vi "Load EEPROM Data.vi"(8 "error in (no error)":errorcluster, 11 "State-machine Local Variables":T1={"Message"="", "Homed?"=FALSE, "NextState"=enum."Timeout", "G.Load"=0.0, "G.Position"=0.0, "Load#"=0, "[G.Loads]"=[], "[TotalLoads]"=[], "[Errors]"=[], "ZeroWait"=0, "Results"=[], "DwellWait"=FALSE, "Test Result"=FALSE, "[CondyleLoads]"=[], "[Max]"=[], "[Min]"=[], "Valid String?"=FALSE, "ScanTime"=timestamp(0 s since 1904-01-01), "ScannedString"="", "LabelDevID"=0, "MfgDate"=timestamp(0 s since 1904-01-01), "[EEPROM Cmds]"=[], "[CalData]"=[], "[A/Ds]"=[], "[A/Dmax]"=[], "[A/Dmin]"=[], "BattMax"=0.0, "BattMin"=0.0, "DwellTime"=2000, "PendingDeviceType"="", "Zero G.load"=0.0, "GAINC Value"="", "Programming Step"=enum."Load EEPROM", "Front Panel Program?"=FALSE, "Final Program?"=FALSE, "PCB Score"=100, "AssyScore"=100, "Pass/Fail #"="", "Result String"="", "Programming Mode"=enum."Initial Program", "Angle Test Step"=enum."Initialize", "Accel Values"=[], "Shutdown Counter"=0, "V1"=0, "V2"=0, "V3"=0, "V4"=0, "EEPROM Data"=[], "Counter"=0, "Page#"=0, "Timer"=timestamp(0 s since 1904-01-01), "Use Mark10?"=FALSE, "Eng-Result#"=0, "DUT Serial #"=0, "Scroll Message?"=FALSE, "Clear Message"=FALSE, "Batt Test Step "=enum."Initialize", "RXTX Window Found?"=FALSE, "Shutdown First Call?"=FALSE, "A2 Delay (msec)"=500, "Support Script"={"Script #"="", "Script Revision"="", "[OEMs]"=[], "[[DeviceTypes]]"=[], "[[DeviceTypesVals]]"=[], "[[List of Errors]]"=[], "Default GAINC"="", "[[ASICtrims]]"=[], "ID For Echo"="", "Condyle A CalFactor"=100, "Condyle B CalFactor"=100, "[OEMs Prefix]"=[], "Packet ID 18"="", "[[Force Table Load Test]]"=[], "[[Force Table AccurTest]]"=[]}, "Serial Table"={"Serial File Path"=path "", "[[Serial Lookup Table]]"=[], "Serial Device Info"=[], "Valid Serial?"=FALSE}, "Target Information"={"Target Brand"="", "Target DeviceType"="", "Target Serial#"=100, "Target Lot#"=0, "Target DevID"=0, "Target Channel"=5}, "Operator"="", "COM Port"="", "Config Path"=path "", "Tx Array"=[], "DUT Parameters"={"Channel"=0, "DeviceID"=0, "Script Rev"=0, "Month"=0, "Day"=0, "Year"=0, "Lot#"=0, "V1"=0, "V2"=0, "V3"=0, "V4"=0, "MFG"=0, "Cal FactorA 10"=0, "Cal FactorB 10  "=0, "Cal FactorA 16"=0, "Cal FactorB 16"=0, "ASICtrim"=[], "TmpChan"=0, "GAINC"="", "Brand"="", "Device"="", "Serial #"=0, "Batt310"=0, "Batt 280"=0}, "FTS Main?"=FALSE, "Loading"={"[Forces]"=[], "[Dwell]"=[], "Loading Step"=enum."Initialize Test"}, "Software Version"="", "Correction Factor"="", "Second Load Test"=FALSE, "Acc Loads"=[], "Mark10 Config"={"H2S%"=[80.0, 85.0, 90.0, 95.0, 100.0], "H2S Speed"=[12.0, 8.0, 6.0, 4.0, 2.0], "H to S"=2.0, "Home Speed"=1.0, "LoadWin"=0.0, "Load Speed"=0.0, "PID"={"Kp"=0.04, "Kd"=0.005001, "Ki"=2.9999999999999923e-05}}, "Channels"={"Transceiver Ch"=5, "Operating Ch"=5, "Start Ch"=0}, "Channel EEPROM"=[], "Load Notes"=[], "Engr Log?"=FALSE, "Time"=[], "Program Retry"=FALSE, "Operator Channel"="", "Target Channel "="", "New Data Program"=FALSE, "NFHU Pass?"=FALSE, "Cycle Number"=0, "Cal Cycle#"=0, "[Avg G.Loads] "=[], "[Avg A/Ds] "=[], "Cal Retry?"=FALSE, "[Total A/Ds]  "=[], "Cycle Num LA"=0, "LA Cycle# "=0, "Shim Num"=0, "Shim#  "=0, "Angle Test?"=FALSE} {"Mark10 Config"."PID"."Ki" min=0.0 max=200.0 format="%.6f"; "Mark10 Config"."PID"."Kd" min=0.0 max=200.0 format="%.6f"; "Mark10 Config"."PID"."Kp" min=0.0 max=200.0 format="%.6f"; "DUT Parameters"."ASICtrim" format="%02x"}) -> (0 "error out":errorcluster, 3 "EEPROM data":u8[][](array[numeric]) format="%02x")   [LabVIEW 2015]
uses:
  Controls/LocalVars.ctl
  Controls/Gen2 FT states.ctl
  Controls/Iniial Device Programming.ctl
  SubVI/ProgramStageControl.ctl
  Controls/Batt Cap Steps.ctl
  Controls/Support Script.ctl
  Controls/Serial Table.ctl
  Controls/Device Information.ctl
  Controls/InfoPacket.ctl
  Controls/Loading.ctl
  Controls/Load Step.ctl
  Controls/Mark10 Config.ctl
  Controls/PID parameters.ctl
  Controls/Channels.ctl
  Controls/DevEEPROMstates.ctl
  <vilib>/Utility/NIReport.llb/NI_report.lvclass
  <vilib>/addons/_office/excel.llb/Excel Get Data ([str]).vi
  <vilib>/addons/_office/NI_ReportGenerationToolkit.lvlib
  <vilib>/Utility/NIReport.llb/Excel/NI_Excel.lvclass
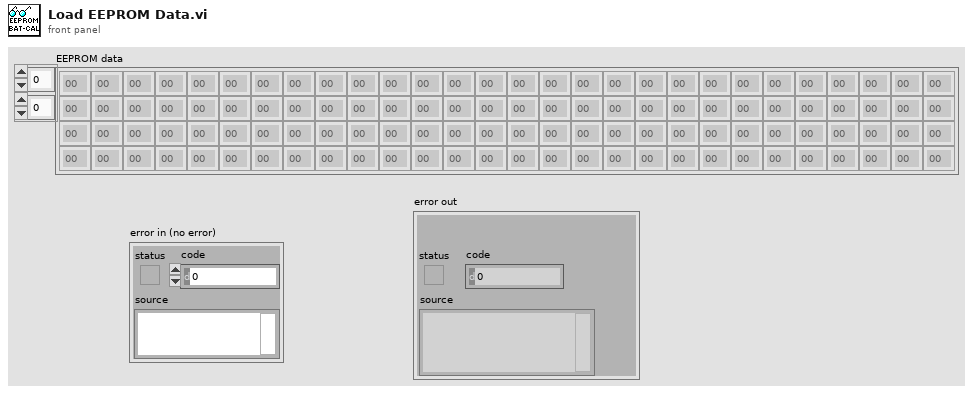
[diagram p1: front panel]
types:
  T1 = typedef "LocalVars.ctl" = cluster{"Message":string, "Homed?":bool, "NextState":T2, "G.Load":dbl, "G.Position":dbl, "Load#":i32, "[G.Loads]":dbl[], "[TotalLoads]":dbl[], "[Errors]":dbl[][], "ZeroWait":u32, "Results":dbl[], "DwellWait":bool, "Test Result":bool, "[CondyleLoads]":dbl[][], "[Max]":dbl[], "[Min]":dbl[], "Valid String?":bool, "ScanTime":timestamp, "ScannedString":string, "LabelDevID":u32, "MfgDate":timestamp, "[EEPROM Cmds]":u8[][], "[CalData]":u8[][], "[A/Ds]":dbl[][], "[A/Dmax]":dbl[], "[A/Dmin]":dbl[], "BattMax":dbl, "BattMin":dbl, "DwellTime":i32, "PendingDeviceType":string, "Zero G.load":dbl, "GAINC Value":string, "Programming Step":T3, "Front Panel Program?":bool, "Final Program?":bool, "PCB Score":i32, "AssyScore":i32, "Pass/Fail #":string, "Result String":string, "Programming Mode":T4, "Angle Test Step":enum16{"Initialize", "Get X", "Get Y", "Get Z", "Next Test"}, "Accel Values":dbl[][], "Shutdown Counter":u32, "V1":i32, "V2":i32, "V3":i32, "V4":i32, "EEPROM Data":i32[][], "Counter":i32, "Page#":i32, "Timer":timestamp, "Use Mark10?":bool, "Eng-Result#":u32, "DUT Serial #":i32, "Scroll Message?":bool, "Clear Message":bool, "Batt Test Step ":T5, "RXTX Window Found?":bool, "Shutdown First Call?":bool, "A2 Delay (msec)":i16, "Support Script":T6, "Serial Table":T7, "Target Information":T8, "Operator":string, "COM Port":string, "Config Path":path, "Tx Array":u8[], "DUT Parameters":T9, "FTS Main?":bool, "Loading":T10, "Software Version":string, "Correction Factor":string, "Second Load Test":bool, "Acc Loads":dbl[][], "Mark10 Config":T12, "Channels":T14, "Channel EEPROM":i32[][], "Load Notes":string[], "Engr Log?":bool, "Time":timestamp[], "Program Retry":bool, "Operator Channel":string, "Target Channel ":string, "New Data Program":bool, "NFHU Pass?":bool, "Cycle Number":i32, "Cal Cycle#":i32, "[Avg G.Loads] ":dbl[], "[Avg A/Ds] ":dbl[][], "Cal Retry?":bool, "[Total A/Ds]  ":dbl[][], "Cycle Num LA":i32, "LA Cycle# ":i32, "Shim Num":i32, "Shim#  ":i32, "Angle Test?":bool}
  T2 = typedef "Gen2 FT states.ctl" = enum16{"---------SETUP-------", "Initialization", "Read Support Data", "Initialize Mark-10", "Initialize Transceiver", "------UTILITIES------", "Change DUT Channel", "Find RxTx Window", "Reset Device", "Scan Channels", "Read Serial Lookup", "Shutdown Device", "ESTOP", "--------USER---------", "Timeout", "-----PROGRAM-----", "Program Device", "------MARK10--------", "Go Home", "MoveUp", "MoveDown", "Goto Load", "Goto Position", "Stop Motor", "---------TESTS--------", "Start Test", "Angle Test", "Load Test", "Load Accuracy Test", "Battery Test", "------RESULTS-------", "End Test", "Display Result", "--------EXIT--------", "Exit"}
  T3 = typedef "Iniial Device Programming.ctl" = enum16{"Load EEPROM", "Send First A1", "Send EEPROM", "Send A1", "Check EEPROM Echo", "Verify transmission", "Programming Successful", "Programming Failed"}
  T4 = typedef "ProgramStageControl.ctl" = enum16{"Initial Program", "GainC", "Scales"}
  T5 = typedef "Batt Cap Steps.ctl" = enum16{"Initialize", "Collect 2.8 Volts", "Collect 3.1 Volts", "Check Results"}
  T6 = typedef "Support Script.ctl" = cluster{"Script #":string, "Script Revision":string, "[OEMs]":string[], "[[DeviceTypes]]":string[][], "[[DeviceTypesVals]]":u16[][], "[[List of Errors]]":string[][], "Default GAINC":string, "[[ASICtrims]]":u8[][], "ID For Echo":string, "Condyle A CalFactor":i32, "Condyle B CalFactor":i32, "[OEMs Prefix]":string[], "Packet ID 18":string, "[[Force Table Load Test]]":dbl[][], "[[Force Table AccurTest]]":dbl[][]}
  T7 = typedef "Serial Table.ctl" = cluster{"Serial File Path":path, "[[Serial Lookup Table]]":string[][], "Serial Device Info":string[], "Valid Serial?":bool}
  T8 = typedef "Device Information.ctl" = cluster{"Target Brand":string, "Target DeviceType":string, "Target Serial#":i32, "Target Lot#":u32, "Target DevID":u32, "Target Channel":u8}
  T9 = typedef "InfoPacket.ctl" = cluster{"Channel":u8, "DeviceID":u32, "Script Rev":u8, "Month":u8, "Day":u8, "Year":u8, "Lot#":u32, "V1":u16, "V2":u16, "V3":u16, "V4":u16, "MFG":u8, "Cal FactorA 10":u8, "Cal FactorB 10  ":u8, "Cal FactorA 16":u8, "Cal FactorB 16":u8, "ASICtrim":u8[], "TmpChan":u8, "GAINC":string, "Brand":string, "Device":string, "Serial #":u64, "Batt310":u16, "Batt 280":u16}
  T10 = typedef "Loading.ctl" = cluster{"[Forces]":dbl[], "[Dwell]":dbl[], "Loading Step":T11}
  T11 = typedef "Load Step.ctl" = enum16{"Initialize Test", "Go Home", "Detect Dev Surface", "Wait to zero Device", "Zero Device", "Do Test", "Test Result"}
  T12 = typedef "Mark10 Config.ctl" = cluster{"H2S%":dbl[], "H2S Speed":dbl[], "H to S":dbl, "Home Speed":dbl, "LoadWin":dbl, "Load Speed":dbl, "PID":T13}
  T13 = typedef "PID parameters.ctl" = cluster{"Kp":dbl, "Kd":dbl, "Ki":dbl}
  T14 = typedef "Channels.ctl" = cluster{"Transceiver Ch":u8, "Operating Ch":u8, "Start Ch":u8}
  T15 = typedef "DevEEPROMstates.ctl" = enum16{"Open Template", "Setup parameters", "Inject parameters", "Read EEPROM data", "Close Template"}
  T16 = enum16{"maximized", "minimized", "normal", "no change"}
  T17 = enum16{"Standard Report", "HTML", "Word", "Excel"}
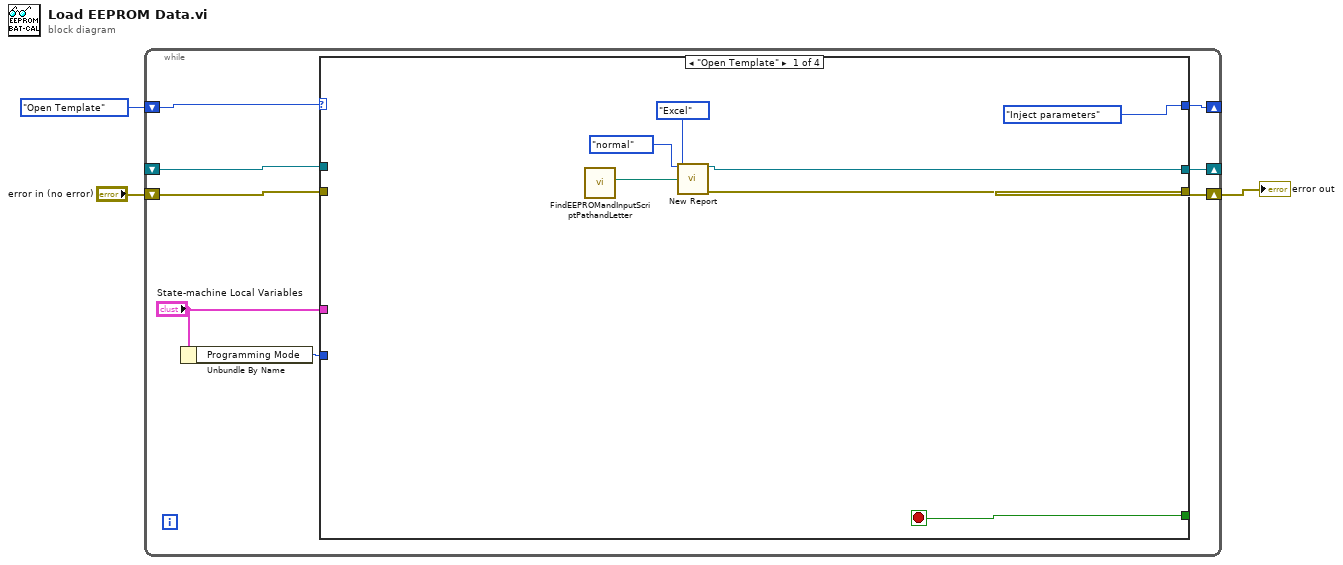
[diagram p0: block diagram]
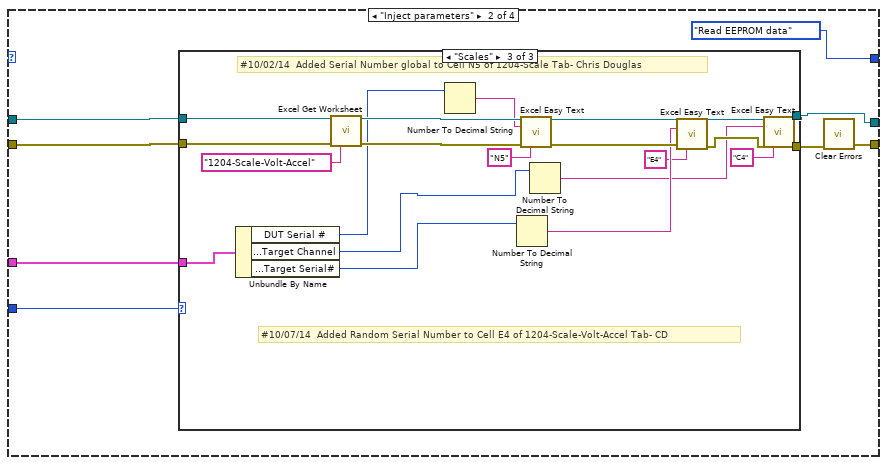
[diagram p2: hidden frame]
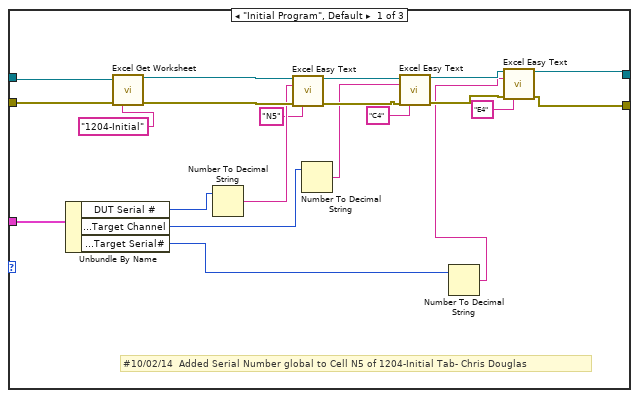
[diagram p3: hidden frame]
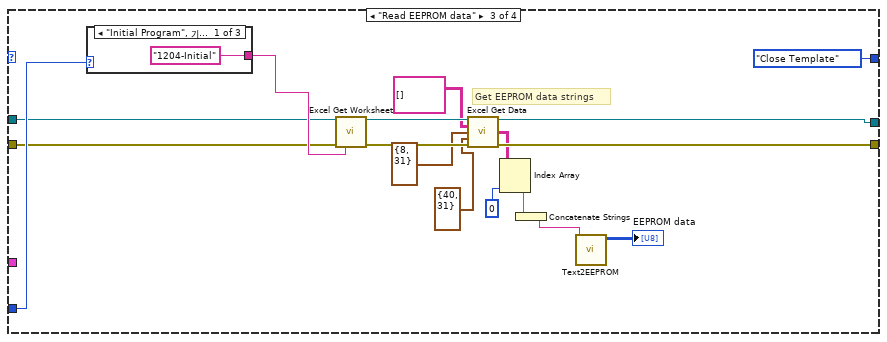
[diagram p5: hidden frame]
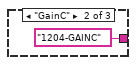
[diagram p6: hidden frame]
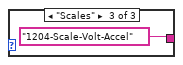
[diagram p7: hidden frame]
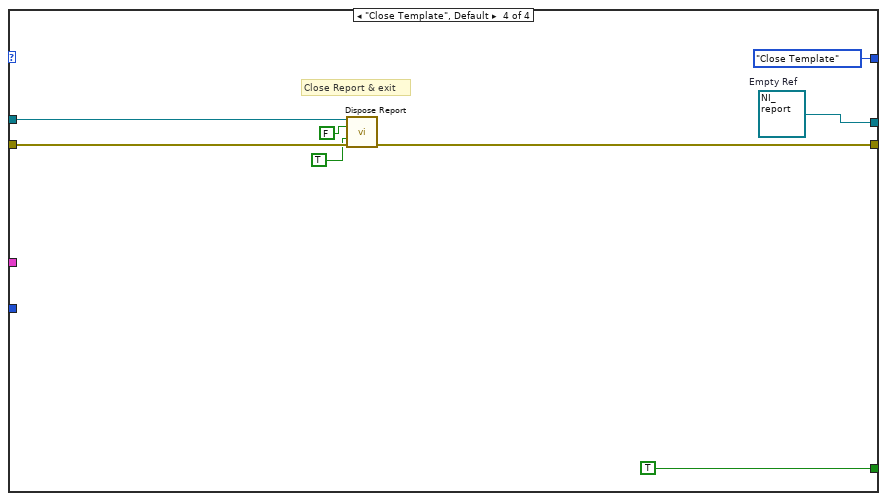
[diagram p8: hidden frame]
diagram:
  n1 = while {
    shift-right: [w4] -> _
    shift-left: _ -> [w11]
    shift-right: [w10] -> w2
    shift-left: "error in (no error)" -> [w9]
    shift-right: [w5] -> _
    shift-left: DevEEPROMstates."Open Template" -> [w8]
    stop <- w12 stop-if-true
    n2 = Unbundle By Name("State-machine Local Variables") -> ("Programming Mode"=w7:T4)
    n3 = case shown="\"Open Template\"" w8 {
      tunnel: [_ _ _ TRUE] -> w12
      tunnel: w11 -> [_ w26 w74 w97]
      tunnel: [w17 w24 w84 w95] -> w10
      tunnel: w9 -> [_ w25 w73 w96]
      tunnel: w7 -> [_ w22 w78 _]
      tunnel: "State-machine Local Variables" -> [_ w21 _ _]
      tunnel: [DevEEPROMstates."Inject parameters" DevEEPROMstates."Read EEPROM data" DevEEPROMstates."Close Template" DevEEPROMstates."Close Template"] -> w5
      tunnel: [w13 w19 w71 w91] -> w4
      frame "Open Template" {
        n4 = call "FindEEPROMandInputScriptPathandLetter.vi"() -> ("Engr Result Path"=w15:path)  [unwired: 7 in, 2 out]
        n5 = call <vilib>:"New Report.vi"("window state (normal)"=T16."normal", "report type"=T17."Excel", "template (empty)"=w15) -> ("report out"=w13:refnum<class "NI_report.lvclass">, "error out"=w17:errorcluster)  [unwired: 11 in]
      }
      frame "Inject parameters" {
        n6 = case shown="\"Scales\"" w22 {
          tunnel: w26 -> [w45 w49 w65]
          tunnel: w25 -> [w44 w48 w64]
          tunnel: [w29 w49 w55] -> w19
          tunnel: [w28 w48 w56] -> w23
          tunnel: w21 -> [w36 _ w53]
          frame "Initial Program", Default {
            # "#10/02/14  Added Serial Number global to Cell N5 of 1204-Initial Tab- Chris Douglas"
            n7 = Unbundle By Name(w36) -> ("DUT Serial #"=w34:i32, "Target Information.Target Channel"=w35:u8, "Target Information.Target Serial#"=w27:i32)
            n8 = call <vilib>:"Excel Get Worksheet.vi"("report in"=w45, "error in (no error)"=w44, "name (\"\")"="1204-Initial" ("name (\"\")")) -> ("report out"=w47:refnum<class "NI_report.lvclass">, "error out"=w46:errorcluster)  [unwired: 11 in]
            n9 = Number To Decimal String(number=w34) -> (decimal integer string=w42:string)  [unwired: 1 in]
            n10 = call <vilib>:"Excel Easy Text.vi"("report in"=w47, "text"=w42, "error in (no error)"=w46, "name (\"\")"="N5" ("name (\"\")")) -> ("report out"=w38:refnum<class "NI_report.lvclass">, "error out"=w39:errorcluster)  [unwired: 7 in, 3 out]
            n11 = Number To Decimal String(number=w35) -> (decimal integer string=w37:string)  [unwired: 1 in]
            n12 = call <vilib>:"Excel Easy Text.vi"("report in"=w38, "text"=w37, "error in (no error)"=w39, "name (\"\")"="C4" ("name (\"\")")) -> ("report out"=w32:refnum<class "NI_report.lvclass">, "error out"=w31:errorcluster)  [unwired: 7 in, 3 out]
            n13 = Number To Decimal String(number=w27) -> (decimal integer string=w30:string)  [unwired: 1 in]
            n14 = call <vilib>:"Excel Easy Text.vi"("report in"=w32, "text"=w30, "error in (no error)"=w31, "name (\"\")"="E4" ("name (\"\")")) -> ("report out"=w29:refnum<class "NI_report.lvclass">, "error out"=w28:errorcluster)  [unwired: 7 in, 3 out]
          }
          frame "GainC" {
          }
          frame "Scales" {
            # "#10/07/14  Added Random Serial Number to Cell E4 of 1204-Scale-Volt-Accel Tab- CD"
            # "#10/02/14  Added Serial Number global to Cell N5 of 1204-Scale Tab- Chris Douglas"
            n15 = Unbundle By Name(w53) -> ("DUT Serial #"=w51:i32, "Target Information.Target Channel"=w52:u8, "Target Information.Target Serial#"=w50:i32)
            n16 = call <vilib>:"Excel Get Worksheet.vi"("report in"=w65, "error in (no error)"=w64, "name (\"\")"="1204-Scale-Volt-Accel" ("name (\"\")")) -> ("report out"=w70:refnum<class "NI_report.lvclass">, "error out"=w69:errorcluster)  [unwired: 11 in]
            n17 = Number To Decimal String(number=w51) -> (decimal integer string=w67:string)  [unwired: 1 in]
            n18 = Number To Decimal String(number=w50) -> (decimal integer string=w61:string)  [unwired: 1 in]
            n19 = call <vilib>:"Excel Easy Text.vi"("report in"=w70, "text"=w67, "error in (no error)"=w69, "name (\"\")"="N5" ("name (\"\")")) -> ("report out"=w63:refnum<class "NI_report.lvclass">, "error out"=w62:errorcluster)  [unwired: 7 in, 3 out]
            n20 = Number To Decimal String(number=w52) -> (decimal integer string=w54:string)  [unwired: 1 in]
            n21 = call <vilib>:"Excel Easy Text.vi"("report in"=w63, "text"=w61, "error in (no error)"=w62, "name (\"\")"="E4" ("name (\"\")")) -> ("report out"=w58:refnum<class "NI_report.lvclass">, "error out"=w57:errorcluster)  [unwired: 7 in, 3 out]
            n22 = call <vilib>:"Excel Easy Text.vi"("report in"=w58, "text"=w54, "error in (no error)"=w57, "name (\"\")"="C4" ("name (\"\")")) -> ("report out"=w55:refnum<class "NI_report.lvclass">, "error out"=w56:errorcluster)  [unwired: 7 in, 3 out]
          }
        }
        n23 = call <vilib>:"Clear Errors.vi"("error in (no error)"=w23) -> ("error out"=w24:errorcluster)  [unwired: 5 in, 1 out]
      }
      frame "Read EEPROM data" {
        # "Get EEPROM data strings"
        n24 = case shown="\"Initial Program\", 기본" w78 {
          tunnel: ["1204-Initial" ("name (\"\")") "1204-GAINC" ("name (\"\")") "1204-Scale-Volt-Accel" ("name (\"\")")] -> w77
          frame "Initial Program", Default {
          }
          frame "GainC" {
          }
          frame "Scales" {
          }
        }
        n25 = call <vilib>:"Excel Get Worksheet.vi"("report in"=w74, "error in (no error)"=w73, "name (\"\")"=w77) -> ("report out"=w86:refnum<class "NI_report.lvclass">, "error out"=w87:errorcluster)  [unwired: 11 in]
        n26 = call-poly <vilib>:"Excel Get Data.vi"("report in"=w86, "data type"=string[][] [], "start (-1, -1)"=cluster{"row":i32, "column":i32} {"row"=8, "column"=31}, "end (-1, -1)"=cluster{"row":i32, "column":i32} {"row"=40, "column"=31}, "error in (no error)"=w87) -> ("report out"=w71:refnum<class "NI_report.lvclass">, "data"=w80:string[][], "error out"=w84:errorcluster)  [unwired: 8 in]
        n27 = Index Array(array=w80, index (col)=0 ("disabled index (col)")) -> (element=w83:string[])  [unwired: 1 in]
        n28 = Concatenate Strings(w83) -> (w82:string)
        n29 = call "Text2EEPROM.vi"("EEPROM Data"=w82) -> ("EEPROM data"=→"EEPROM data":u8[][])  [unwired: 10 in]
      }
      frame "Close Template", Default {
        w91 = refnum<class "NI_report.lvclass"> refnum  # Empty Ref
        # "Close Report & exit"
        n30 = call-dynamic "Dispose Report.vi"("report in"=w97, "wait until printing completed? (T)"=FALSE, "save changes? (F)"=TRUE, "error in (no error)"=w96) -> ("error out"=w95:errorcluster)  [unwired: 11 in]
      }
    }
  }
  "error out" <- w2
